vi "polyDistort_apn.vi"(8 "error in (no error)":errorcluster, 9 "Backward?":bool=TRUE, 10 "polyIn":dbl[](array[numeric]), 11 "lineDataIn":sgl[](array[numeric])) -> (0 "error out":errorcluster, 3 "distoredDataOut":dbl[](array[numeric]) format="%_6g")   [LabVIEW 2016]
uses:
  <vilib>/Analysis/polynomials.llb/1D Polynomial Evaluation (DBL).vi
  <vilib>/Analysis/NI_AALPro.lvlib
  <vilib>/gmath/NI_Gmath.lvlib
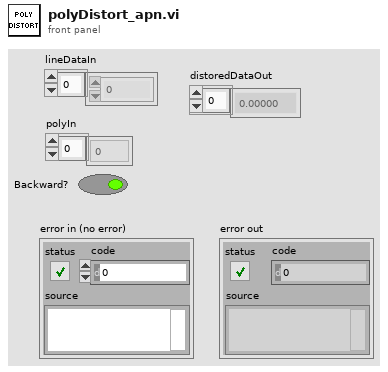
[diagram p1: front panel]
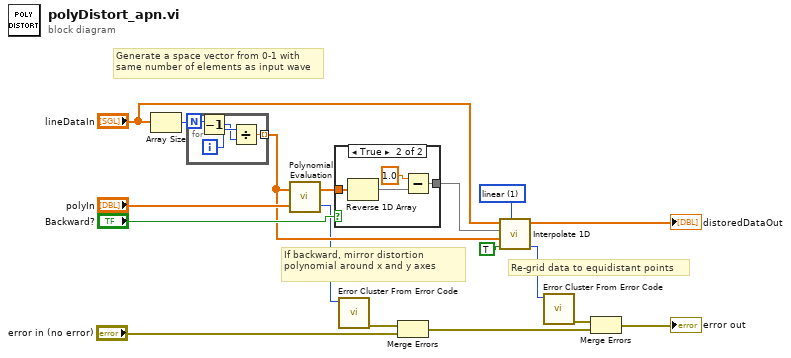
[diagram p0: block diagram]
diagram:
  w13 = 1 items=["nearest", "linear", "spline", "cubic Hermite", "Lagrange"] ("method")
  # "Generate a space vector from 0-1 with same number of elements as input wave"
  # "Re-grid data to equidistant points"
  # "If backward, mirror distortion polynomial around x and y axes"
  n1 = Array Size(array="lineDataIn") -> (size(s)=w17:i32)
  n2 = for {
    N: w17 -> [w20]
    tunnel: [w19] -> w11 mode=indexing
    i -> [w21]
    n3 = Decrement(x=w20) -> (x-1=w18:i32)
    n4 = Divide(x=w21, y=w18) -> (x/y=w19:dbl)
  }
  n5 = call-poly <vilib>:"Polynomial Evaluation.vi"("P(x)"="polyIn", "A"=w11) -> ("error"=w7:i32, "P(A)"=w14:dbl[])
  n6 = case shown="True" "Backward?" {
    tunnel: w14 -> [w22 w26]
    tunnel: [w22 w23] -> w12
    frame False {
    }
    frame True {
      n7 = Reverse 1D Array(array=w26) -> (reversed array=w24:dbl[])
      n8 = Subtract(x=1.0, y=w24) -> (x-y=w23:dbl[])
    }
  }
  n9 = call <vilib>:"Error Cluster From Error Code.vi"("error code (0)"=w7) -> ("error out"=w6:errorcluster)  [unwired: 8 in]
  n10 = Merge Errors(w6, "error in (no error)") -> (w2:errorcluster)
  n11 = call <vilib>:"Interpolate 1D.vi"("method"=w13, "X is monotonic"=TRUE, "xi"=w11, "X"=w12, "Y"="lineDataIn") -> ("error"=w4:i32, "yi"=→"distoredDataOut":dbl[])  [unwired: 4 in, 1 out]
  n12 = call <vilib>:"Error Cluster From Error Code.vi"("error code (0)"=w4) -> ("error out"=w3:errorcluster)  [unwired: 8 in]
  n13 = Merge Errors(w3, w2) -> (→"error out":errorcluster)
